vi "Ref To Library.vi"(8 "error in (no error)":errorcluster, 11 "ProjectItem in":refnum<vi>) -> (0 "error out":errorcluster, 3 "Library out":refnum<vi>)   [LabVIEW 2019, in "gRPC Template Creation Utility.lvlib"]
uses:
  gRPC Template Creation Utility.lvlib
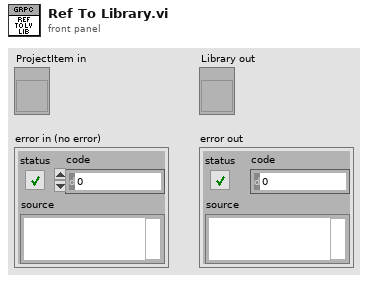
[diagram p1: front panel]
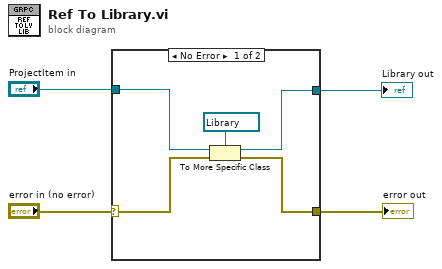
[diagram p0: block diagram]
diagram:
  n1 = case shown="No Error" "error in (no error)" {
    selector: "error in (no error)" -> [w5 w10]
    tunnel: [w9 _] -> w4
    tunnel: [w8 w10] -> w3
    tunnel: "ProjectItem in" -> [w7 _]
    frame No Error {
      n2 = To More Specific Class(target class=refnum<vi> refnum ("Library out"), reference=w7, error in=w5) -> (specific class reference=w9:refnum<vi>, error out=w8:errorcluster)
    }
    frame Error {
    }
  }
  "Library out" <- w4
  "error out" <- w3
